vi "Text Changed.vi"(8 "error in (no error)":errorcluster, 10 "Text":string, 11 "Text Message in":refnum<class "Text Message.lvclass">) -> (0 "error out":errorcluster, 3 "Text Message out":refnum<class "Text Message.lvclass">)   [LabVIEW 2011, in "Text Message.lvclass"]
uses:
  Text Message.lvclass
  Observable/Observable.lvclass
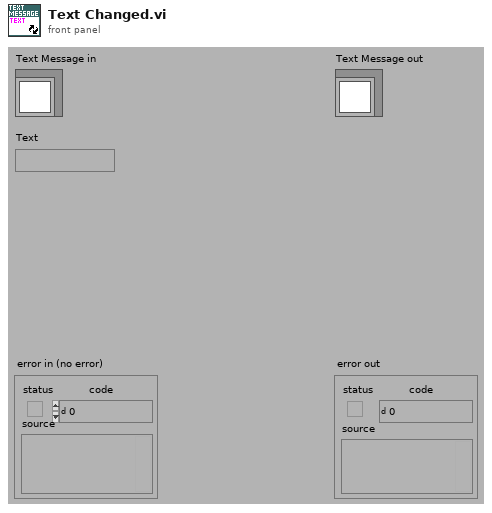
[diagram p1: front panel]
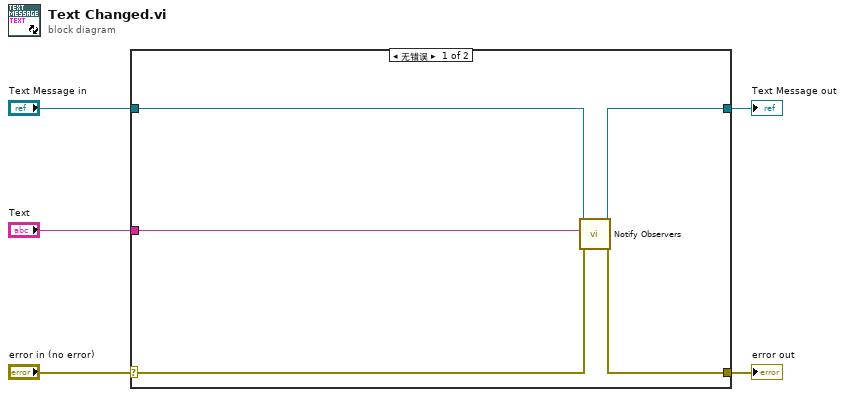
[diagram p0: block diagram]
diagram:
  n1 = case shown="无错误" "error in (no error)" {
    selector: "error in (no error)" -> [w7 w12]
    tunnel: [w9 w12] -> w2
    tunnel: [w10 w11] -> w4
    tunnel: "Text Message in" -> [w8 w11]
    tunnel: "Text" -> [w6 _]
    frame No Error {
      n2 = call "Notify Observers.vi"("error in (no error)"=w7, "Text"=w6, "Observable in"=w8) -> ("error out"=w9:errorcluster, "Observable out"=w10:refnum<class "Text Message.lvclass">)  [unwired: 7 in]
    }
    frame Error {
    }
  }
  "Text Message out" <- w4
  "error out" <- w2
